vi "Set PID.vi"(5 "Output #":i32=1, 6 "D":dbl, 7 "P manual":dbl, 8 "error in (no error)":errorcluster, 9 "I":dbl, 10 "P":dbl, 11 "LakeShore T Controller Driver in":refnum<class "LakeShore T Controller Driver.lvclass">) -> (0 "error out":errorcluster, 3 "LakeShore T Controller Driver out":refnum<class "LakeShore T Controller Driver.lvclass">)   [LabVIEW 2021, in "LakeShore T Controller Driver.lvclass"]
uses:
  LakeShore T Controller Driver.lvclass
  LakeShore T Controller Driver.lvclass/LakeShore T Controller Driver.ctl
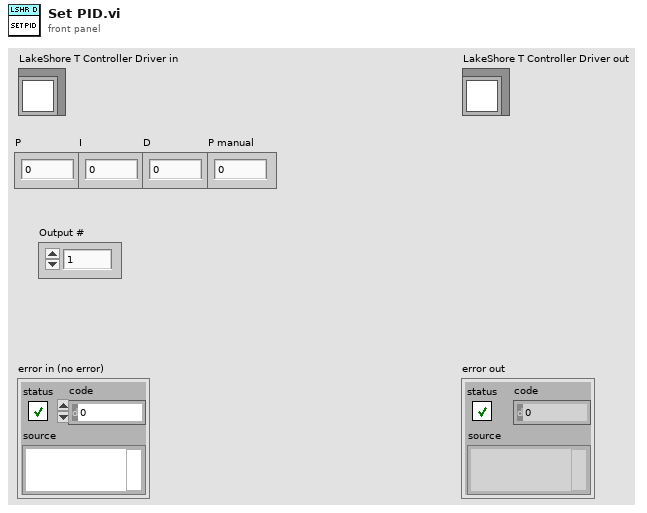
[diagram p1: front panel]
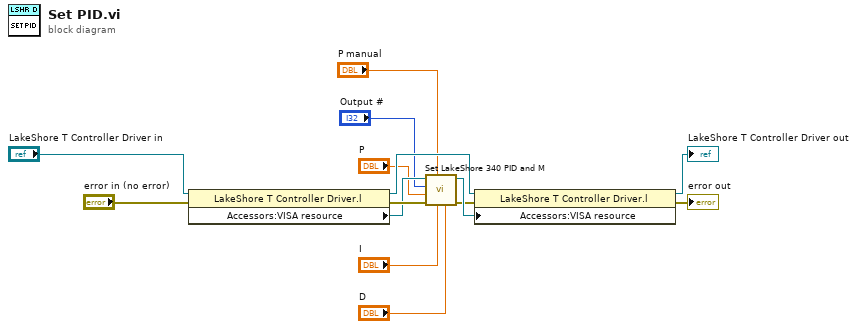
[diagram p0: block diagram]
diagram:
  n1 = property class="LakeShore T Controller Driver.l"(reference="LakeShore T Controller Driver in", error in="error in (no error)") -> (reference out=w11:refnum<class "LakeShore T Controller Driver.lvclass">, error out=w13:errorcluster, "Accessors:VISA resource"=w12:refnum<visa-resource-name>)
  n2 = call "Set LakeShore 340 PID and M.vi"("D"="D", "I"="I", "Manual otput"="P manual", "error in (no error)"=w13, "P"="P", "Output #"="Output #", "VISA Resource Name"=w12) -> ("error out"=w1:errorcluster, "VISA Resource Name Out"=w2:refnum<visa-resource-name>)  [unwired: 3 in]
  n3 = property class="LakeShore T Controller Driver.l"(reference=w11, error in=w1, "Accessors:VISA resource"=w2) -> (reference out=→"LakeShore T Controller Driver out":refnum<class "LakeShore T Controller Driver.lvclass">, error out=→"error out":errorcluster)
